vi "Map Channels to Doubles.vi"(10 "register values":u16[](array[numeric]) format="%x", 11 "Channel Data":T1[](array[typedef])) -> (3 "Array":dbl[](array[numeric]))   [LabVIEW 2021, in "Modbus Master Engine.lvlib"]
uses:
  Modbus Master Engine.lvlib
  Shared/Controls/Data Model/Channel.ctl
  System Explorer/SubVIs/Modbus Type.ctl
  <vilib>/NI VeriStand/Custom Device API/Custom Device Channel Type.ctl
  Shared/Controls/Data Model/Mapping.ctl
  Shared/Controls/Data Model/DataType.ctl
  <vilib>/NI VeriStand/Custom Device API/Custom Device Item Ref.ctl
  Shared/Modbus Master Shared.lvlib
  <vilib>/NI VeriStand/Custom Device API/Custom Device API.lvlib
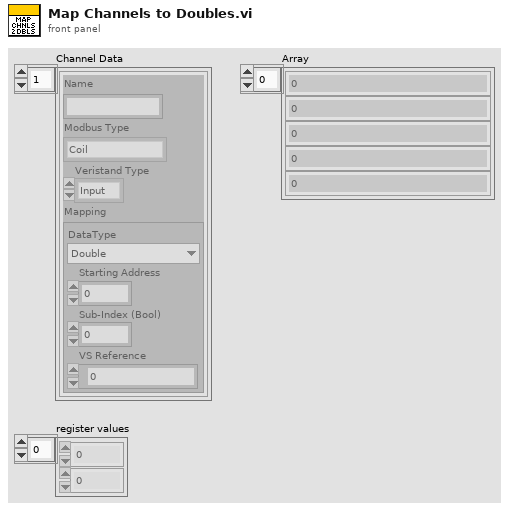
[diagram p1: front panel]
types:
  T1 = typedef "Modbus Master Shared.lvlib/Channel.ctl" = cluster{"Name":string, "Modbus Type":T2, "Veristand Type":T3, "Mapping":T4}
  T2 = typedef "Modbus Master Shared.lvlib/Modbus Type.ctl" = enum16{"Coil", "Discrete Input", "Holding Register", "Input Register"}
  T3 = typedef "Custom Device API.lvlib/Custom Device Channel Type.ctl" = enum16{"Input", "Output"}
  T4 = typedef "Modbus Master Shared.lvlib/Mapping.ctl" = cluster{"DataType":T5, "Starting Address":u16, "Sub-Index (Bool)":u16, "VS Reference":T6}
  T5 = typedef "Modbus Master Shared.lvlib/DataType.ctl" = enum16{"Double", "Single", "I64", "I32", "I16", "I8", "U64", "U32", "U16", "U8", "Boolean"}
  T6 = typedef "Custom Device API.lvlib/Custom Device Item Ref.ctl" = u64
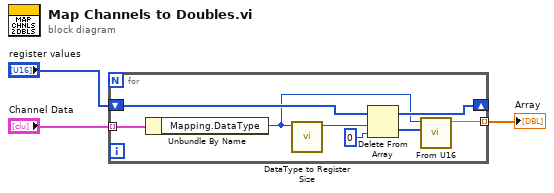
[diagram p0: block diagram]
diagram:
  n1 = for {
    tunnel: "Channel Data" -> [w11] mode=indexing
    shift-right: [w9] -> _
    shift-left: "register values" -> [w10]
    tunnel: [w4] -> w3 mode=indexing
    n2 = Unbundle By Name(w11) -> ("Mapping.DataType"=w6:T5)
    n3 = call "DataType to Register Size.vi"("DataType"=w6) -> ("Registers"=w7:i32)  [unwired: 9 in, 1 out]
    n4 = Delete From Array(array=w10, length=w7, index=0) -> (deleted portion=w5:u16[], array with subset deleted=w9:u16[])
    n5 = call "From U16.vi"("Array"=w5, "DataType"=w6) -> ("Numeric"=w4:dbl)  [unwired: 9 in]
  }
  "Array" <- w3
